vi "Encoder2Postition_Translation.vi"(10 "Signal from Encoder":dbl, 11 "Initial Position":dbl) -> (3 "Postion Trans":dbl)   [LabVIEW 2019]
panel:
  # "This Vi calculates from the encoder signal the absolut translational position in [mm]."
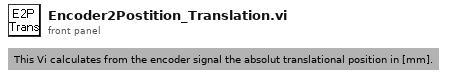
[diagram p1: front panel]
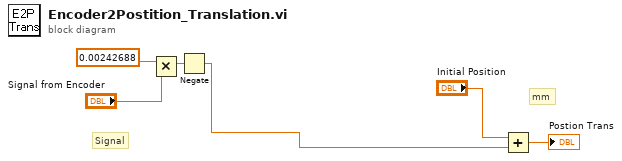
[diagram p0: block diagram]
diagram:
  # "mm"
  # "Signal"
  n1 = Multiply(x=0.00242688, y="Signal from Encoder") -> (x*y=w4:dbl)
  n2 = Negate(x=w4) -> (-x=w1:dbl)
  n3 = Add(x="Initial Position", y=w1) -> (x+y=→"Postion Trans":dbl)
